vi "isNumber.vi"(8 "error in (no error)":errorcluster, 10 "string":string, 11 "CommandParser in":refnum<class "CommandParser.lvclass">) -> (0 "error out":errorcluster, 2 "isNumber?":bool, 3 "CommandParser out":refnum<class "CommandParser.lvclass">)   [LabVIEW 2016, in "CommandParser.lvclass"]
uses:
  CommandParser.lvclass
  <vilib>/regexp/Match Regular Expression.xnode
panel:
  out "after match":string
  out "whole match":string
  out "before match":string
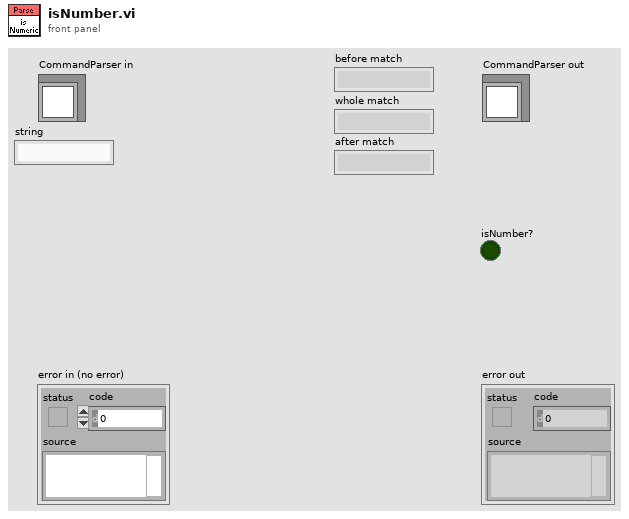
[diagram p1: front panel]
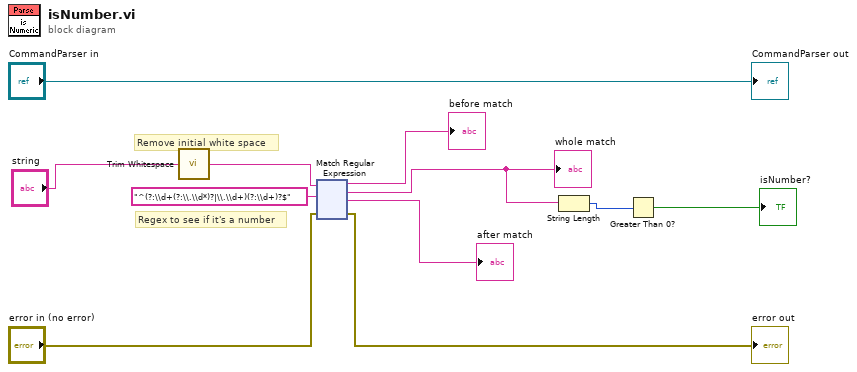
[diagram p0: block diagram]
diagram:
  # "Regex to see if it's a number"
  # "Remove initial white space"
  n1 = call <vilib>:"Trim Whitespace.vi"("string"="string") -> ("trimmed string"=w1:string)  [unwired: 1 in]
  n2 = xnode "Match Regular Expression"("input string"=w1, "regular expression"="^(?:\\d+(?:\\.\\d*)?|\\.\\d+)(?:\\d+)?$", "error in"="error in (no error)") -> ("before match"=→"before match":string, "whole match"=w5:string, "after match"=→"after match":string, "error out"=→"error out":errorcluster)  [unwired: 3 in, 1 out]
  "whole match" <- w5
  n3 = String Length(string=w5) -> (length=w4:i32)
  n4 = Greater Than 0?(x=w4) -> (x > 0?=→"isNumber?":bool)
  "CommandParser out" <- "CommandParser in"
